vi "Read Notifier Map.vi"(8 "error in (no error)":errorcluster, 11 "Simiple Map SEQ 64 Notifier Controller Factory in":refnum<class "Simiple Map Notifier Controller Factory.lvclass">) -> (0 "error out":errorcluster, 2 "Notifier Map":map{i64, refnum<class "Notifier.lvclass">}(c390), 3 "Simiple Map SEQ 64 Notifier Controller Factory out":refnum<class "Simiple Map Notifier Controller Factory.lvclass">)   [LabVIEW 2024, in "Simiple Map Notifier Controller Factory.lvclass"]
uses:
  Simiple Map Notifier Controller Factory.lvclass
  Ancestor Class/Actor Assistant/Notifier/Notifier.lvclass
  Simiple Map Notifier Controller Factory.lvclass/Simiple Map Notifier Controller Factory.ctl
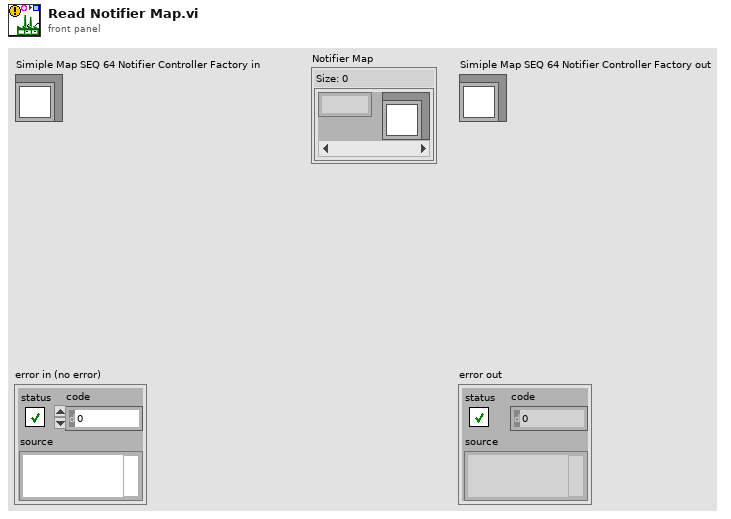
[diagram p1: front panel]
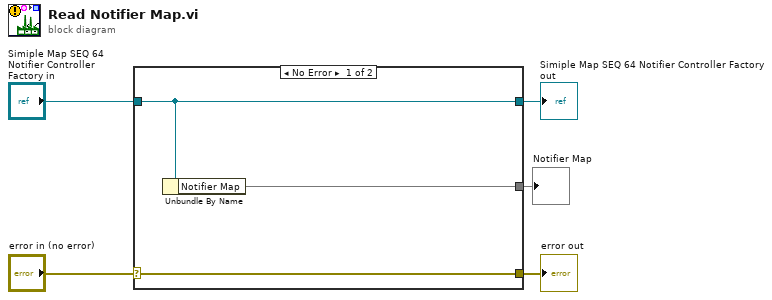
[diagram p0: block diagram]
diagram:
  n1 = case shown="No Error" "error in (no error)" {
    selector: "error in (no error)" -> [w8 w9]
    tunnel: [w8 w9] -> w4
    tunnel: [w7 w10] -> w2
    tunnel: "Simiple Map SEQ 64 Notifier Controller Factory in" -> [w7 w10]
    tunnel: [w6 _] -> w1
    frame No Error {
      n2 = Unbundle By Name(w7) -> ("Notifier Map"=w6:map{i64, refnum<class "Notifier.lvclass">})
    }
    frame Error {
    }
  }
  "error out" <- w4
  "Simiple Map SEQ 64 Notifier Controller Factory out" <- w2
  "Notifier Map" <- w1
